vi "Extract Auto Sequence Data.vi"(7 "Data Cluster":T1, 8 "error in (no error)":errorcluster, 9 "Cancellled?":bool, 10 "Exists?":bool, 11 "Folder Path":path) -> (0 "error out":errorcluster, 5 "Data Cluster Out":T1)   [LabVIEW 2021, in "Test Configuration.lvlib"]
uses:
  Test Configuration.lvlib
  Module Data--cluster.ctl
  Host-Control's/Module ID Action Enum.ctl
  Host-Control's/HW Name Enum.ctl
  <vilib>/Utility/xml.llb/Read From XML File.vi
  <vilib>/Utility/xml.llb/Read From XML File(string).vi
panel:
  out "filename without extension":string
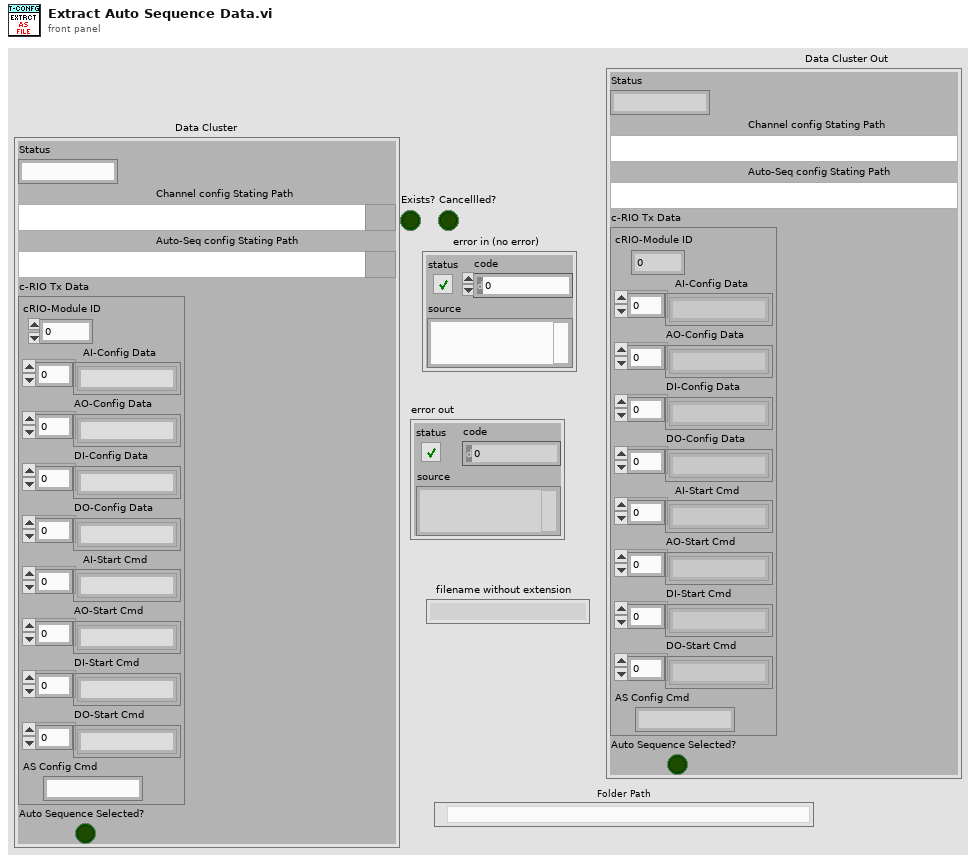
[diagram p1: front panel]
types:
  T1 = typedef "Test Configuration.lvlib/Module Data--cluster.ctl" = cluster{"Status":string, "Channel config Stating Path":path, "Auto-Seq config Stating Path":path, "c-RIO Tx Data":cluster{"cRIO-Module ID":i32, "AI-Config Data":string[], "AO-Config Data":string[], "DI-Config Data":string[], "DO-Config Data":string[], "AI-Start Cmd":string[], "AO-Start Cmd":string[], "DI-Start Cmd":string[], "DO-Start Cmd":string[], "AS Config Cmd":string}, "Auto Sequence Selected?":bool}
  T2 = typedef "HW Name Enum.ctl" = enum16{"Capsule-1", "Capsule-2", "Capsule-3", "Capsule-4", "sb-RIO", "Safety", "Release"}
  T3 = typedef "Module ID Action Enum.ctl" = enum16{"Init", "Insert", "Get a ID", "Get all ID"}
  T4 = cluster{"Select Channel":bool, "Physical Channel Name":string, "Identification Name":string, "  Start\nOn/Off":bool, "Start Time":dbl, "  End\nOn/Off":bool, "End Time (S)":dbl}[]
  T5 = cluster{"Physical Channel Name":string, "Identification Name":string, "Operation":bool, "Time":dbl}[]
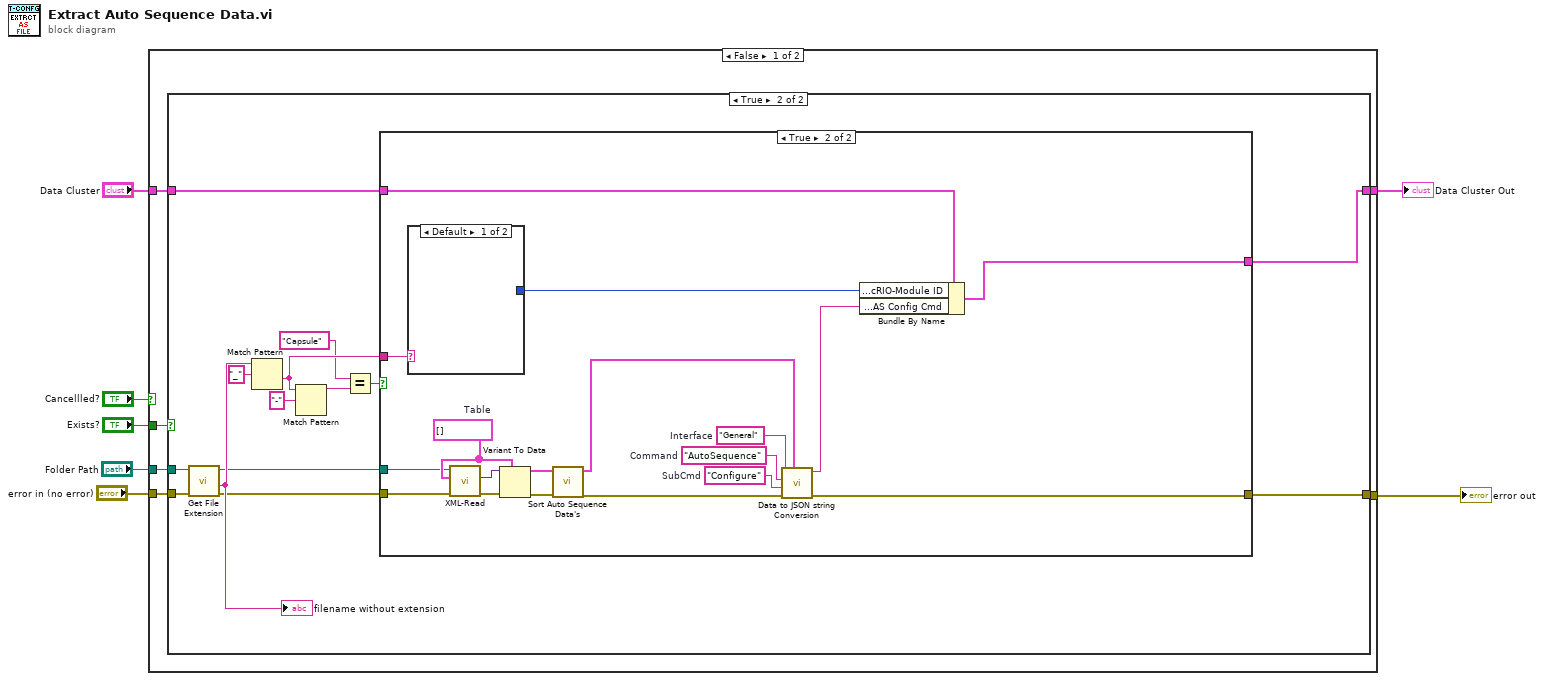
[diagram p0: block diagram]
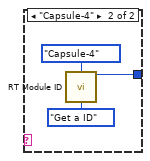
[diagram p4: hidden frame]
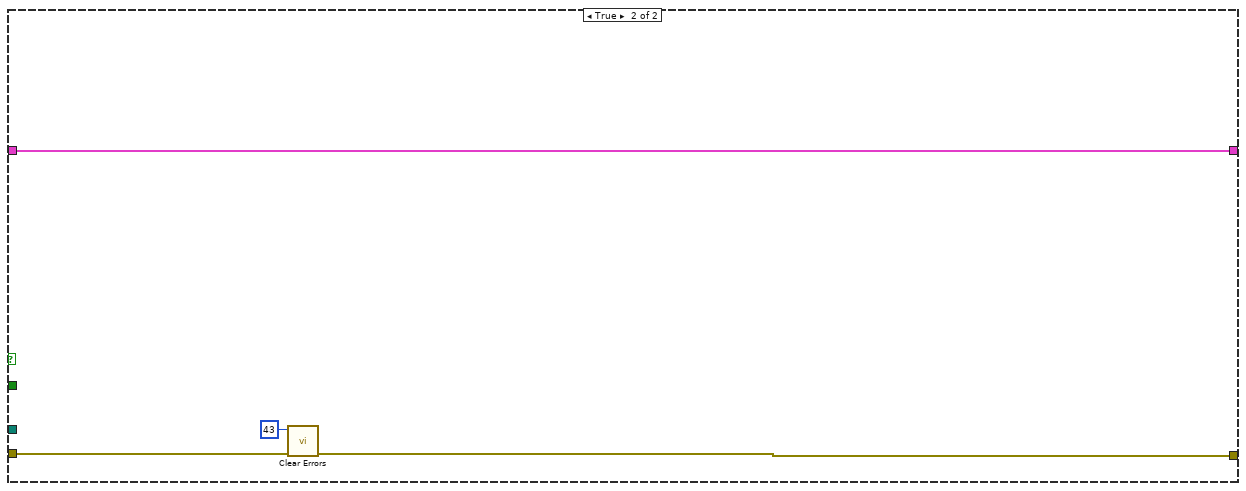
[diagram p5: hidden frame]
diagram:
  n1 = case shown="False" "Cancellled?" {
    tunnel: "error in (no error)" -> [w13 w55]
    tunnel: [w12 w54] -> w2
    tunnel: "Folder Path" -> [w10 _]
    tunnel: "Exists?" -> [w11 _]
    tunnel: "Data Cluster" -> [w9 w56]
    tunnel: [w8 w56] -> w3
    frame False {
      n2 = case shown="True" w11 {
        tunnel: w13 -> [w15 w28]
        tunnel: [w15 w16] -> w12
        tunnel: w10 -> [_ w29]
        tunnel: w9 -> [w14 w27]
        tunnel: [w14 w22] -> w8
        frame False {
        }
        frame True {
          n3 = call <vilib>:"Get File Extension.vi"("error in (no error)"=w28, "file"=w29) -> ("error out"=w24:errorcluster, "filename without extension"=w25:string, "dup file"=w23:path)  [unwired: 5 in, 2 out]
          "filename without extension" <- w25
          n4 = Match Pattern(string=w25, regular expression="_") -> (after substring=w21:string)  [unwired: 1 in, 3 out]
          n5 = Match Pattern(string=w21, regular expression="-") -> (before substring=w18:string)  [unwired: 1 in, 3 out]
          n6 = Equal?(x="Capsule" ("before substring"), y=w18) -> (x = y?=w17:bool)
          n7 = case shown="True" w17 {
            tunnel: w27 -> [w31 w49]
            tunnel: w24 -> [w30 w32]
            tunnel: w23 -> [_ w35]
            tunnel: [w31 w44] -> w22
            tunnel: w21 -> [_ w43]
            tunnel: [w30 w38] -> w16
            frame False {
            }
            frame True {
              w48 = "Configure"  # SubCmd
              w47 = "AutoSequence"  # Command
              w46 = "General"  # Interface
              w36 = T4 []  # Table
              n8 = case shown="Default" w43 {
                tunnel: [_ w50] -> w45
                frame Default {
                }
                frame "Capsule-4" {
                  n9 = call "RT Module ID.vi"("HW Name"=HW_Name_Enum."Capsule-4", "Action"=Module_ID_Action_Enum."Get a ID") -> ("Module Id Out"=w50:i32)  [unwired: 10 in, 3 out]
                }
              }
              n10 = call "XML-Read.vi"("error in (no error)"=w32, "Data"=w36, "XML File Path"=w35) -> ("error out"=w33:errorcluster, "Data Out"=w34:variant)  [unwired: 6 in, 1 out]
              n11 = Variant To Data(error in=w33, type=w36, Variant=w34) -> (data=w41:T4, error out=w40:errorcluster)
              n12 = call "Sort Auto Sequence Data's.vi"("error in (no error)"=w40, "Table"=w41) -> ("error out"=w39:errorcluster, "Sorted AS Data"=w37:T5)  [unwired: 8 in]
              n13 = call "Data to JSON string Conversion.vi"("Data"=w37, "error in"=w39, "SubCmd"=w48, "Command"=w47, "Interface"=w46) -> ("error out"=w38:errorcluster, "Cmd String"=w42:string)  [unwired: 5 in]
              n14 = Bundle By Name(cluster=w49, "c-RIO Tx Data.cRIO-Module ID"=w45, "c-RIO Tx Data.AS Config Cmd"=w42) -> (w44:T1)
            }
          }
        }
      }
    }
    frame True {
      n15 = call <vilib>:"Clear Errors.vi"("error in (no error)"=w55, "specific error code to clear (0: all)"=43) -> ("error out"=w54:errorcluster)  [unwired: 4 in, 1 out]
    }
  }
  "Data Cluster Out" <- w3
  "error out" <- w2
